vi "GetEnableAndPOCStatusChDataRef.vi"(8 "error in":errorcluster, 11 "Device Reference in":T2 format="%.0x") -> (0 "error out":errorcluster, 2 "Channel Data Refs":T1[](array[typedef]) format="%.0x", 3 "Device Ref out":T2 format="%.0x")   [LabVIEW 2020, in "FlexRay Custom Device Engine.lvlib"]
uses:
  FlexRay Custom Device Engine.lvlib
  <vilib>/NI VeriStand/Custom Device API/Custom Device Item Ref.ctl
  <vilib>/NI VeriStand/Custom Device API/Data Reference.ctl
  <vilib>/NI VeriStand/Custom Device API/Data Access Type.ctl
  <vilib>/NI VeriStand/Custom Device API/Custom Device API.lvlib
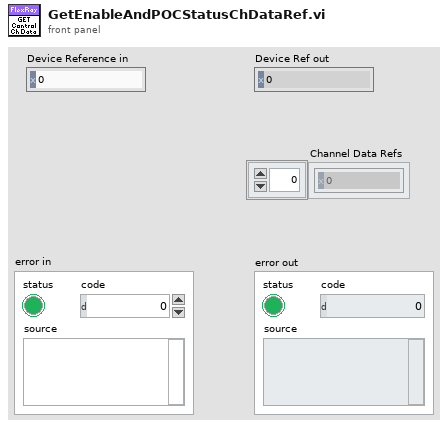
[diagram p1: front panel]
types:
  T1 = typedef "Custom Device API.lvlib/Data Reference.ctl" = i32
  T2 = typedef "Custom Device API.lvlib/Custom Device Item Ref.ctl" = u64
  T3 = typedef "Custom Device API.lvlib/Data Access Type.ctl" = enum16{"Read", "Write"}
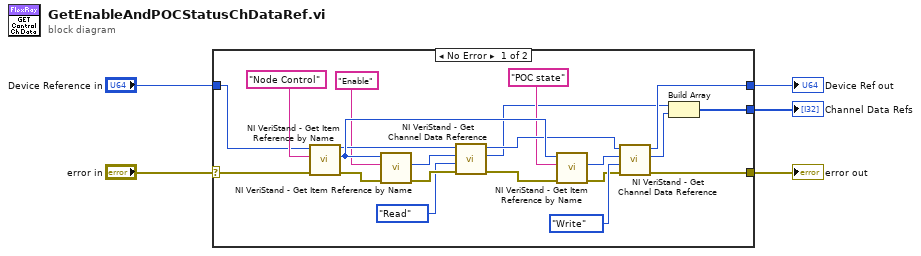
[diagram p0: block diagram]
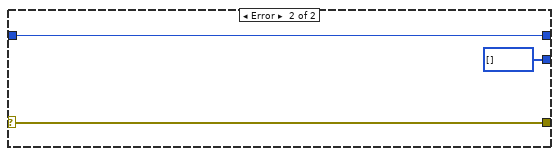
[diagram p2: hidden frame]
diagram:
  n1 = case shown="No Error" "error in" {
    selector: "error in" -> [w6 w29]
    tunnel: [w23 w28] -> w5
    tunnel: "Device Reference in" -> [w9 w28]
    tunnel: [w8 T1[] []] -> w3
    tunnel: [w7 w29] -> w2
    frame No Error {
      n2 = call <vilib>:"NI VeriStand - Get Item Reference by Name.vi"("error in (no error)"=w6, "Item Name"="Node Control" ("Section Name"), "Parent Ref in"=w9) -> ("error out"=w14:errorcluster, "Item Ref"=w24:T2, "Parent Ref out"=w16:T2)  [unwired: 5 in, 1 out]
      n3 = call <vilib>:"NI VeriStand - Get Item Reference by Name.vi"("error in (no error)"=w14, "Item Name"="Enable" ("Channel Name"), "Parent Ref in"=w24) -> ("error out"=w15:errorcluster, "Item Ref"=w12:T2)  [unwired: 5 in, 2 out]
      n4 = call <vilib>:"NI VeriStand - Get Channel Data Reference.vi"("error in (no error)"=w15, "Access"=Data_Access_Type."Read", "Channel Ref in"=w12, "Device Ref in"=w16) -> ("error out"=w25:errorcluster, "Channel Data Reference"=w17:T1, "Device Ref out"=w22:T2)  [unwired: 5 in]
      n5 = call <vilib>:"NI VeriStand - Get Item Reference by Name.vi"("error in (no error)"=w25, "Item Name"="POC state" ("Channel Name"), "Parent Ref in"=w24) -> ("error out"=w18:errorcluster, "Item Ref"=w19:T2)  [unwired: 5 in, 2 out]
      n6 = call <vilib>:"NI VeriStand - Get Channel Data Reference.vi"("error in (no error)"=w18, "Access"=Data_Access_Type."Write", "Channel Ref in"=w19, "Device Ref in"=w22) -> ("error out"=w7:errorcluster, "Channel Data Reference"=w26:T1, "Device Ref out"=w23:T2)  [unwired: 5 in]
      n7 = Build Array(w17, w26) -> (w8:T1[])
    }
    frame Error {
    }
  }
  "Device Ref out" <- w5
  "Channel Data Refs" <- w3
  "error out" <- w2
